vi "Setup Dependencies.vi"(8 "error in (no error)":errorcluster, 10 "Windows Bin File":path, 11 "Item Ref in":T1 format="%.0x") -> (0 "error out":errorcluster)   [LabVIEW 2015, in "AIT 664 Custom Device.lvlib"]
uses:
  AIT 664 Custom Device.lvlib
  <vilib>/NI Veristand/Custom Device API/Custom Device Item Ref.ctl
  <vilib>/NI Veristand/Custom Device API/Custom Device Supported Target.ctl
  <vilib>/NI Veristand/Custom Device API/Path Type.ctl
  <vilib>/NI Veristand/Custom Device API/Custom Device File Dependency.ctl
  <vilib>/NI Veristand/Custom Device API/Path Specification.ctl
  <vilib>/NI Veristand/Custom Device API/Custom Device API.lvlib
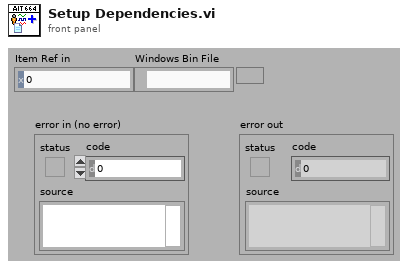
[diagram p1: front panel]
types:
  T1 = typedef "Custom Device API.lvlib/Custom Device Item Ref.ctl" = u64
  T2 = typedef "Custom Device API.lvlib/Custom Device File Dependency.ctl" = cluster{"Source":T3, "RT Destination":path, "ForceDownload?":bool, "SupportedTarget":T5, "Version":string}
  T3 = typedef "Custom Device API.lvlib/Path Specification.ctl" = cluster{"Path":path, "Type":T4}
  T4 = typedef "Custom Device API.lvlib/Path Type.ctl" = enum16{"Absolute", "To Base", "To Common Data Dir", "To Application Data Dir"}
  T5 = typedef "Custom Device API.lvlib/Custom Device Supported Target.ctl" = enum16{"All", "PharLap", "VxWorks", "Windows", "Linux_32_ARM", "Linux_x64", "PharLap & Windows", "PharLap & VxWorks", "VxWorks & Windows"}
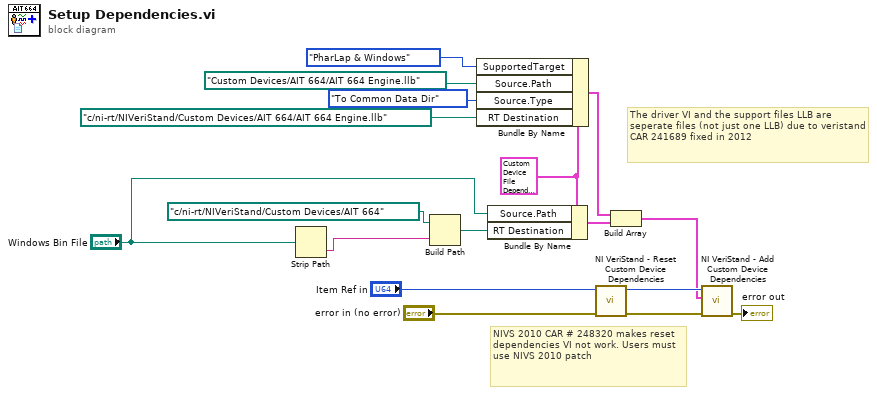
[diagram p0: block diagram]
diagram:
  w11 = T2 {"Source"={"Path"=path "", "Type"=enum."Absolute"}, "RT Destination"=path "c:/ni-rt/NIVeriStand/Custom Devices/AIT 429", "ForceDownload?"=FALSE, "SupportedTarget"=enum."PharLap", "Version"=""} ("Dependency")
  # "The driver VI and the support files LLB are seperate files (not just one LLB) due to veristand CAR 241689 fixed in 2012"
  # "NIVS 2010 CAR # 248320 makes reset dependencies VI not work. Users must use NIVS 2010 patch"
  n1 = Strip Path(path="Windows Bin File") -> (name=w4:string)  [unwired: 1 out]
  n2 = Build Path(base path=path "c:/ni-rt/NIVeriStand/Custom Devices/AIT 664" ("RT Destination"), name or relative path=w4) -> (appended path=w12:path)
  n3 = Bundle By Name(cluster=w11, "SupportedTarget"=Custom_Device_Supported_Target."PharLap & Windows", "Source.Path"=path "Custom Devices/AIT 664/AIT 664 Engine.llb", "Source.Type"=Path_Type."To Common Data Dir", "RT Destination"=path "c:/ni-rt/NIVeriStand/Custom Devices/AIT 664/AIT 664 Engine.llb") -> (w10:T2)
  n4 = Bundle By Name(cluster=w11, "Source.Path"="Windows Bin File", "RT Destination"=w12) -> (w13:T2)
  n5 = call <vilib>:"NI VeriStand - Reset Custom Device Dependencies.vi"("error in (no error)"="error in (no error)", "Device Ref in"="Item Ref in") -> ("error out"=w16:errorcluster, "Device Ref out"=w15:T1)  [unwired: 8 in]
  n6 = Build Array(w10, w13) -> (w14:T2[])
  n7 = call <vilib>:"NI VeriStand - Add Custom Device Dependencies.vi"("error in (no error)"=w16, "Dependencies"=w14, "Device Ref in"=w15) -> ("error out"=→"error out":errorcluster)  [unwired: 7 in, 1 out]
